vi "23.vi"() -> ()   [LabVIEW 2021]
panel:
  out "Array":i32[](array[numeric])
  out "Set":set{i32}(c389)
  out "Numeric":i32
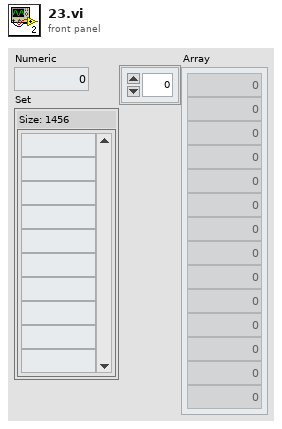
[diagram p1: front panel]
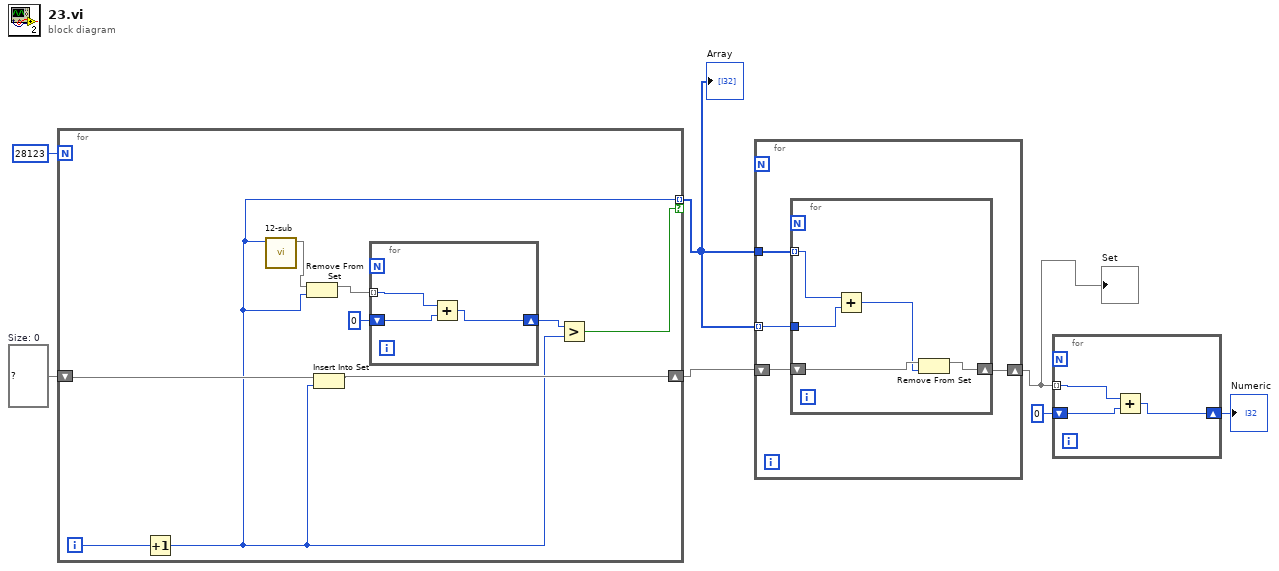
[diagram p0: block diagram]
diagram:
  w6 = set{i32} {}  # Size: 0
  n1 = for {
    N: 28123 -> [_]
    shift-right: [w14] -> w4
    shift-left: w6 -> [w15]
    tunnel: [w8] -> w5 mode=indexing if=w11
    i -> [w16]
    n2 = Increment(x=w16) -> (x+1=w8:i32)
    n3 = call "12-sub.vi"("Number"=w8) -> ("Divisors"=w9:set{i32})  [unwired: 9 in, 1 out]
    n4 = Remove From Set(10:w8, 11:w9) -> (3:w10:set{i32})  [unwired: 1 out]
    n5 = Insert Into Set(10:w8, 11:w15) -> (3:w14:set{i32})  [unwired: 1 out]
    n6 = for {
      tunnel: w10 -> [w19] mode=indexing
      shift-right: [w17] -> w12
      shift-left: 0 -> [w18]
      n7 = Add(x=w19, y=w18) -> (x+y=w17:i32)
    }
    n8 = Greater?(x=w12, y=w8) -> (0:w11:bool)
  }
  "Array" <- w5
  n9 = for {
    tunnel: w5 -> [w23]
    tunnel: w5 -> [w22] mode=indexing
    shift-right: [w21] -> w1
    shift-left: w4 -> [w20]
    n10 = for {
      tunnel: w23 -> [w28] mode=indexing
      tunnel: w22 -> [w27]
      shift-right: [w26] -> w21
      shift-left: w20 -> [w25]
      n11 = Add(x=w28, y=w27) -> (x+y=w24:i32)
      n12 = Remove From Set(10:w24, 11:w25) -> (3:w26:set{i32})  [unwired: 1 out]
    }
  }
  "Set" <- w1
  n13 = for {
    tunnel: w1 -> [w31] mode=indexing
    shift-right: [w29] -> w2
    shift-left: 0 -> [w30]
    n14 = Add(x=w31, y=w30) -> (x+y=w29:i32)
  }
  "Numeric" <- w2
